vi "Get Spare Sensor Channels.vi"(10 "Existing":string[](array[string])) -> (1 "Tasks":refnum<k21>[](array[refnum]), 2 "Spares":string[](array[string]))   [LabVIEW 2013]
uses:
  Metadata/Persistant DAO Actions.ctl
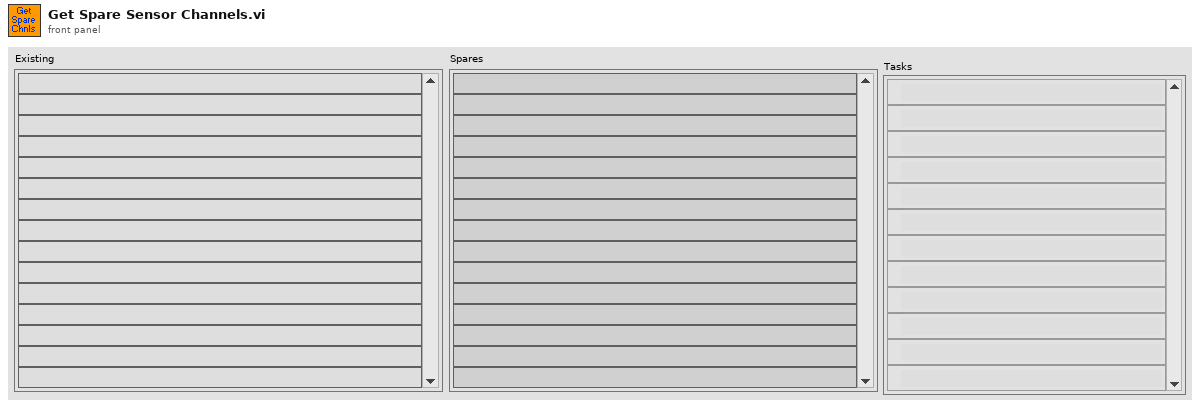
[diagram p1: front panel]
types:
  T1 = typedef "Persistant DAO Actions.ctl" = enum16{"Init", "Get", "Set", "Load", "Save"}
  T2 = typedef "DAQMx Tasks.ctl" = cluster{"LBCB1 Readings":refnum<k21>, "LBCB2 Readings":refnum<k21>, "LBCB1 Commands":refnum<k21>, "LBCB2 Commands":refnum<k21>, "Sensors":refnum<k21>[]}
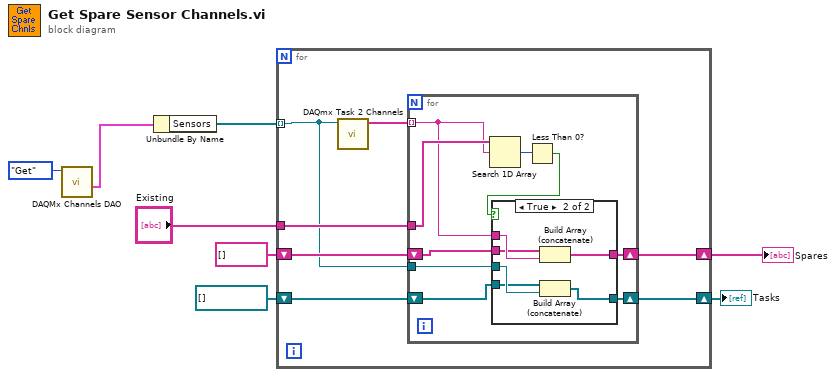
[diagram p0: block diagram]
diagram:
  n1 = call "DAQMx Channels DAO.vi"("Actions"=Persistant_DAO_Actions."Get") -> ("Names Out"=w7:T2)  [unwired: 8 in, 2 out]
  n2 = Unbundle By Name(w7) -> ("Sensors"=w6:refnum<k21>[])
  n3 = for {
    tunnel: w6 -> [w11] mode=indexing
    tunnel: "Existing" -> [w14]
    shift-right: [w13] -> w3
    shift-left: string[] [] -> [w12]
    shift-right: [w10] -> w1
    shift-left: refnum<k21>[] [] -> [w9]
    n4 = call "DAQmx Task 2 Channels.vi"("DAQmx Task Name"=w11) -> ("Channels Out"=w15:string[])  [unwired: 10 in]
    n5 = for {
      tunnel: w15 -> [w21] mode=indexing
      tunnel: w14 -> [w24]
      shift-right: [w20] -> w13
      shift-left: w12 -> [w19]
      tunnel: w11 -> [w18]
      shift-right: [w17] -> w10
      shift-left: w9 -> [w16]
      n6 = Search 1D Array(1D array=w24, element=w21) -> (index of element=w23:i32)  [unwired: 1 in]
      n7 = Less Than 0?(x=w23) -> (x < 0?=w22:bool)
      n8 = case shown="True" w22 {
        tunnel: w21 -> [_ w32]
        tunnel: [w26 w31] -> w20
        tunnel: w19 -> [w26 w30]
        tunnel: w18 -> [_ w29]
        tunnel: [w25 w28] -> w17
        tunnel: w16 -> [w25 w27]
        frame False {
        }
        frame True {
          n9 = Build Array (concatenate)(w30, w32) -> (w31:string[])
          n10 = Build Array (concatenate)(w27, w29) -> (w28:refnum<k21>[])
        }
      }
    }
  }
  "Spares" <- w3
  "Tasks" <- w1
